vi "CreateBroadcasts.vi"(8 "error in (no error)":errorcluster) -> (0 "error out":errorcluster, 3 "StandardBroadcasts":T1)   [LabVIEW 2024, in "RQMHModule.lvclass"]
uses:
  RQMHModule.lvclass
  StandardBroadcasts.ctl
  Shared/Died.ctl
  Started.ctl
  RQMHModule.lvclass/RQMHModule.ctl
  Shared/JQMHShared.lvlib
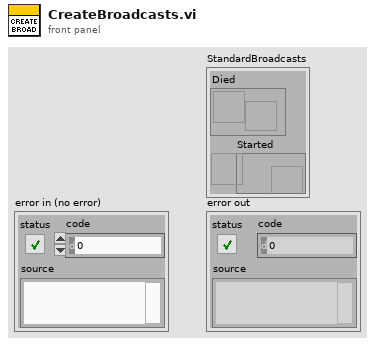
[diagram p1: front panel]
types:
  T1 = typedef "RQMHModule.lvclass/StandardBroadcasts.ctl" = cluster{"Died":refnum<user-event>, "Started":refnum<user-event>}
  T2 = typedef "RQMHModule.lvclass/Started.ctl" = bool
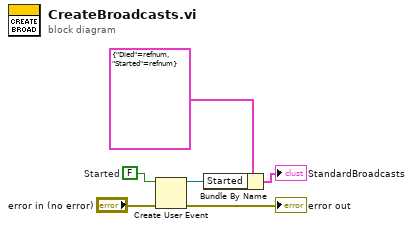
[diagram p0: block diagram]
diagram:
  w3 = T2 FALSE  # Started
  n1 = Create User Event(user event datatype=w3, error in="error in (no error)") -> (user event=w4:refnum<user-event>, error out=→"error out":errorcluster)
  n2 = Bundle By Name(cluster=T1 {"Died"=refnum, "Started"=refnum} ("StandardBroadcasts"), "Started"=w4) -> (→"StandardBroadcasts":T1)
